vi "Set Double Definition.vi"(10 "Double Definition":T1, 11 "Double in":refnum<class "Double.lvclass">) -> (3 "Double out":refnum<class "Double.lvclass">)   [LabVIEW 2020, in "Conditu2.lvlib" / "Columns.lvlib" / "Double.lvclass"]
uses:
  Double.lvclass
  Definition.ctl
  Double.lvclass/Double.ctl
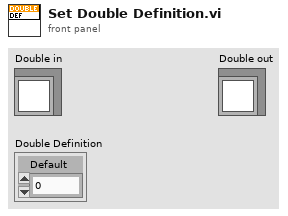
[diagram p1: front panel]
types:
  T1 = typedef "Conditu2.lvlib/Columns.lvlib/Double.lvclass/Definition.ctl" = cluster{"Default":dbl}
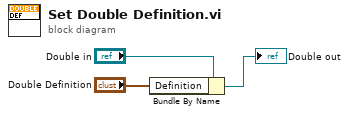
[diagram p0: block diagram]
diagram:
  n1 = Bundle By Name(cluster="Double in", "Definition"="Double Definition") -> (→"Double out":refnum<class "Double.lvclass">)
